vi "set_use.vi"(4 "Remote Server Address":string="palantir", 5 "Listen Port":u16=5311, 6 "Remote Server Port":u16=5310, 7 "error in (no error)":errorcluster, 8 "User":string, 9 "In Use?":bool, 10 "Target Name":string) -> (0 "error out":errorcluster, 2 "success":bool)   [LabVIEW 2011]
uses:
  TCPdata.ctl
  TargetData.ctl
panel:
  in  "Cluster":T1
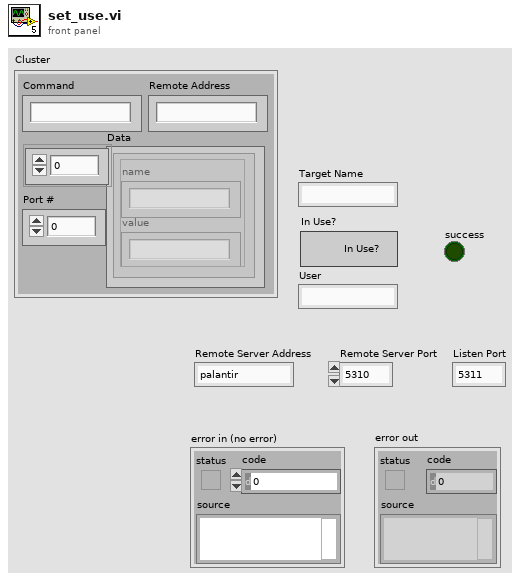
[diagram p1: front panel]
types:
  T1 = typedef "TCPdata.ctl" = cluster{"Data":T2, "Command":string, "Remote Address":string, "Port #":u16}
  T2 = typedef "TargetData.ctl" = cluster{"name":string, "value":string}[]
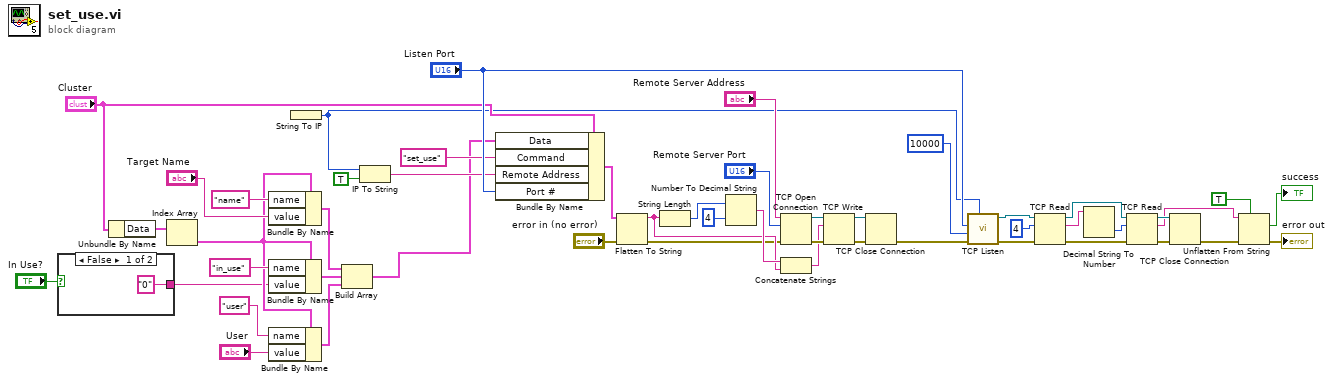
[diagram p0: block diagram]
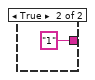
[diagram p2: hidden frame]
diagram:
  n1 = case shown="False" "In Use?" {
    tunnel: ["0" ("value") "1" ("value")] -> w1
    frame False {
    }
    frame True {
    }
  }
  n2 = Unbundle By Name("Cluster") -> ("Data"=w34:T2)
  n3 = Index Array(array=w34) -> (element=w5:cluster{"name":string, "value":string})  [unwired: 1 in]
  n4 = Bundle By Name(cluster=w5, "name"="name", "value"="Target Name") -> (w33:cluster{"name":string, "value":string})
  n5 = Bundle By Name(cluster=w5, "name"="in_use", "value"=w1) -> (w4:cluster{"name":string, "value":string})
  n6 = Bundle By Name(cluster=w5, "name"="user", "value"="User") -> (w3:cluster{"name":string, "value":string})
  n7 = String To IP() -> (0:w29:u32)  [unwired: 1 in]
  n8 = Build Array(w33, w4, w3) -> (w32:cluster{"name":string, "value":string}[])
  n9 = IP To String(1:TRUE ("dot notation? (F)"), 2:w29) -> (0:w37:string)
  n10 = Bundle By Name(cluster="Cluster", "Data"=w32, "Command"="set_use", "Remote Address"=w37, "Port #"="Listen Port") -> (w24:T1)
  n11 = Flatten To String(anything=w24, error in (no error)="error in (no error)") -> (data string=w23:string, error out=w21:errorcluster)  [unwired: 2 in, 1 out]
  n12 = String Length(string=w23) -> (length=w27:i32)
  n13 = Number To Decimal String(number=w27, width (-)=i16 4) -> (decimal integer string=w26:string)
  n14 = TCP Open Connection(address="Remote Server Address", remote port or service name="Remote Server Port", error in (no error)=w21) -> (connection ID=w49:refnum<k5>, error out=w48:errorcluster)  [unwired: 2 out]
  n15 = Concatenate Strings(w26, w23) -> (w28:string)
  n16 = TCP Write(connection ID=w49, data in=w28, error in (no error)=w48) -> (connection ID out=w46:refnum<k5>, error out=w47:errorcluster)  [unwired: 2 out]
  n17 = TCP Close Connection(connection ID=w46, error in (no error)=w47) -> (error out=w40:errorcluster)  [unwired: 2 out]
  n18 = call <vilib>:"TCP Listen.vi"("net address"=w29, "error in (no error)"=w40, "timeout ms (wait forever: -1)"=10000, "port"="Listen Port") -> ("error out"=w18:errorcluster, "connection ID"=w16:refnum<k5>)  [unwired: 3 in, 3 out]
  n19 = TCP Read(connection ID=w16, bytes to read=4, error in (no error)=w18) -> (connection ID out=w15:refnum<k5>, data out=w19:string, error out=w17:errorcluster)  [unwired: 1 in, 1 out]
  n20 = Decimal String To Number(string=w19) -> (number=w14:i32)  [unwired: 2 in, 1 out]
  n21 = TCP Read(connection ID=w15, bytes to read=w14, error in (no error)=w17) -> (connection ID out=w43:refnum<k5>, data out=w12:string, error out=w41:errorcluster)  [unwired: 1 in, 1 out]
  n22 = TCP Close Connection(connection ID=w43, error in (no error)=w41) -> (error out=w13:errorcluster)  [unwired: 2 out]
  n23 = Unflatten From String(type=TRUE, binary string=w12, error in (no error)=w13) -> (value=→"success":bool, error out=→"error out":errorcluster)  [unwired: 2 in, 1 out]
